vi "Read Measurement Name.vi"(8 "error in (no error)":errorcluster, 11 "Measurement in":refnum<class "Function.lvclass">) -> (0 "error out":errorcluster, 2 "Measurement Name":string, 3 "Measurement out":refnum<class "Function.lvclass">)   [LabVIEW 2016, in "Function Actor.lvlib" / "Function.lvclass"]
uses:
  <userlib>/Common Components/Function Actor/Function.lvclass
  <userlib>/Common Components/Function Actor/Function.lvclass/Function.ctl
  <userlib>/_OpenG.lib/file/file.llb/Strip Path Extension - String__ogtk.vi
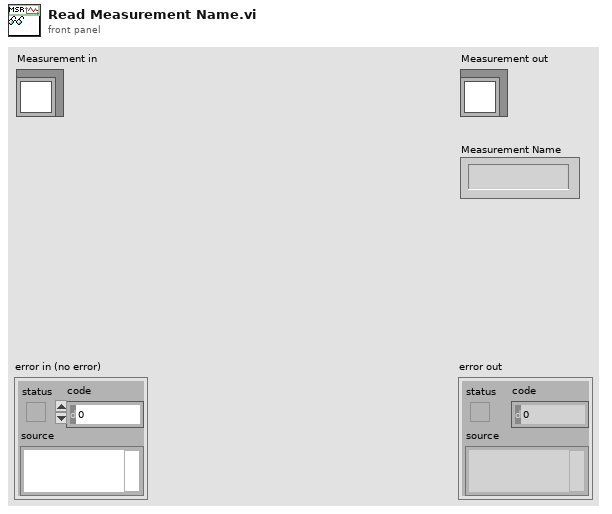
[diagram p1: front panel]
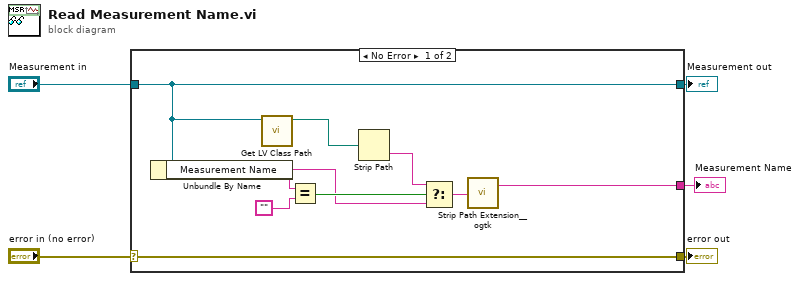
[diagram p0: block diagram]
diagram:
  n1 = case shown="No Error" "error in (no error)" {
    selector: "error in (no error)" -> [w14 w15]
    tunnel: [w14 w15] -> w4
    tunnel: [w10 w16] -> w2
    tunnel: "Measurement in" -> [w10 w16]
    tunnel: [w6 _] -> w1
    frame No Error {
      n2 = Unbundle By Name(w10) -> ("Measurement Name"=w11:string)
      n3 = call <vilib>:"Get LV Class Path.vi"("object"=w10) -> ("class path"=w8:path)  [unwired: 9 in, 1 out]
      n4 = Equal?(x=w11, y="") -> (x = y?=w12:bool)
      n5 = Strip Path(path=w8) -> (name=w9:string)  [unwired: 1 out]
      n6 = Select(t=w9, s=w12, f=w11) -> (s? t:f=w7:string)
      n7 = call-poly <userlib>:"Strip Path Extension__ogtk.vi"("path"=w7) -> ("root"=w6:string)  [unwired: 1 out]
    }
    frame Error {
    }
  }
  "error out" <- w4
  "Measurement out" <- w2
  "Measurement Name" <- w1
